vi "get_x_data_array.vi"(8 "error in (no error)":errorcluster, 11 "Plots in":refnum<class "Plots.lvclass">) -> (0 "error out":errorcluster, 2 "x-Array":dbl[](array[numeric]), 3 "Plots out":refnum<class "Plots.lvclass">)   [LabVIEW 2017, in "Plots.lvclass"]
doc: "returns all of the good (flag =0) x-data as array"
uses:
  Plots.lvclass
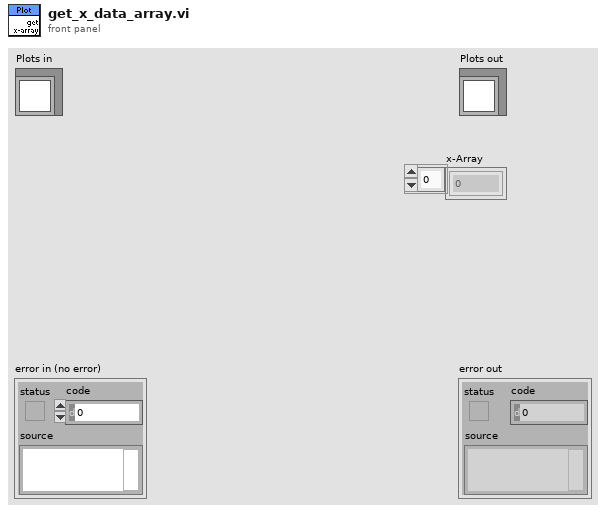
[diagram p1: front panel]
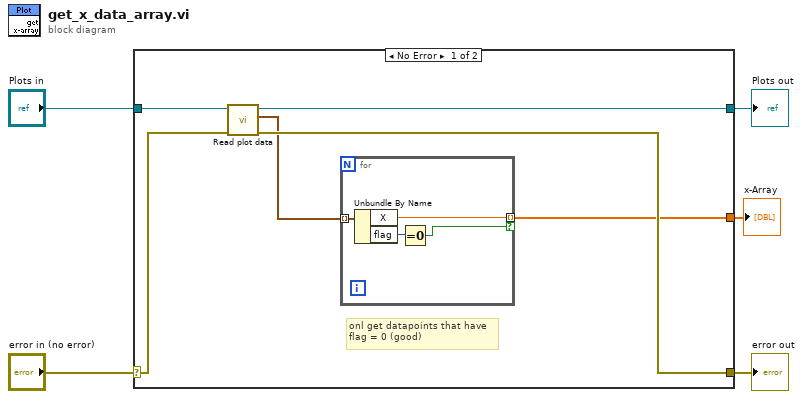
[diagram p0: block diagram]
diagram:
  n1 = case shown="No Error" "error in (no error)" {
    selector: "error in (no error)" -> [w10 w17]
    tunnel: [w9 w17] -> w4
    tunnel: [w8 w16] -> w2
    tunnel: "Plots in" -> [w11 w16]
    tunnel: [w6 _] -> w1
    frame No Error {
      # "onl get datapoints that have\nflag = 0 (good)"
      n2 = call-dynamic "Read plot data.vi"("error in (no error)"=w10, "Plots in"=w11) -> ("error out"=w9:errorcluster, "plot data"=w7:cluster{"X":dbl, "Y":dbl, "flag":u8}[], "Plots out"=w8:refnum<class "Plots.lvclass">)  [unwired: 7 in]
      n3 = for {
        tunnel: w7 -> [w15] mode=indexing
        tunnel: [w14] -> w6 mode=indexing if=w12
        n4 = Unbundle By Name(w15) -> ("X"=w14:dbl, "flag"=w13:u8)
        n5 = Equal To 0?(x=w13) -> (x = 0?=w12:bool)
      }
    }
    frame Error {
    }
  }
  "error out" <- w4
  "Plots out" <- w2
  "x-Array" <- w1
